vi "Apply.vi"(8 "error in":errorcluster, 11 "Camera Config Imaqdx in":refnum<class "Camera Imaqdx CFG.lvclass">) -> (0 "error out":errorcluster, 3 "Camera Config Imaqdx out":refnum<class "Camera Imaqdx CFG.lvclass">)   [LabVIEW 2023, in "Camera Imaqdx CFG.lvclass"]
uses:
  Camera Imaqdx CFG.lvclass
  Camera Imaqdx CFG.lvclass/Camera Imaqdx CFG.ctl
  <resource>/objmgr/imaqdx.rc
  <vilib>/vision/driver/IMAQdx.llb/IMAQdx Attribute Type.ctl
  c47df427-a957-40c2-9a9c-b1ab8804aafe.vi
  c5374de2-410c-459e-aecd-e99eee27f195.vi
  8bc8691d-3ecb-4910-bc1f-a4c379582725.vi
  7010e766-7afd-408f-98f0-f2143d80f09c.vi
  90c98f4d-8272-4d06-bdee-effaadf9e15a.vi
  4e38bbe0-b2bb-4691-89cd-49c1504e38ab.vi
  Configuration Base/Configuration Base.lvclass
  <vilib>/ErrorRing/Error Ring.xnode
  <vilib>/Utility/error.llb/Error Cluster From Error Code.vi
  E:/git/HAL/Configuration Base/Configuration Base.lvclass
  E:/git/HAL/Interfaces/IConfigure/IConfigure.lvclass
  E:/git/HAL/Camera Imaqdx/Configuration/Camera Imaqdx CFG.lvclass
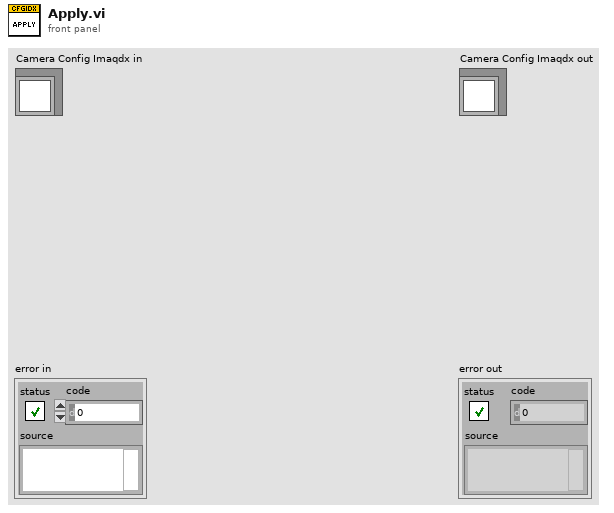
[diagram p1: front panel]
types:
  T1 = typedef "NI_Vision_Acquisition_Software.lvlib/IMAQdx Attribute Type.ctl" = enum32{"U32", "I64", "DBL", "String", "Enum", "Bool", "Command"}
  T2 = typedef "IMAQdx.ctl" = refnum<k21>
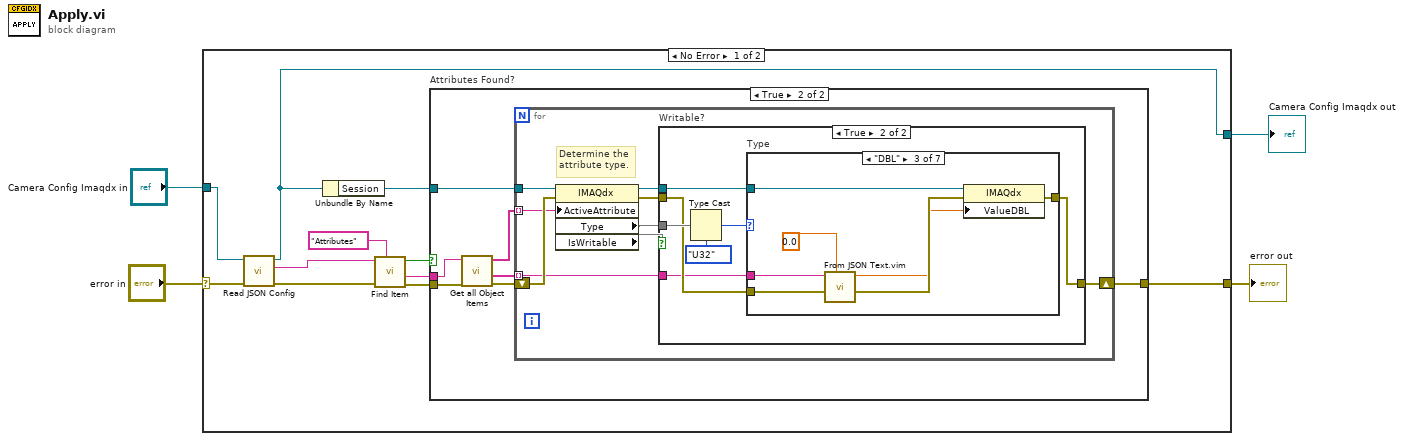
[diagram p0: block diagram]
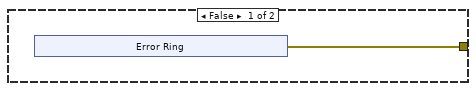
[diagram p2: hidden frame]
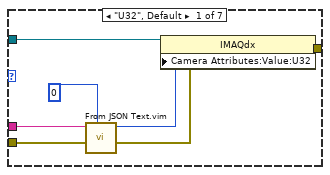
[diagram p4: hidden frame]
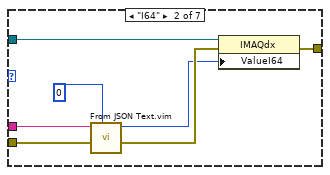
[diagram p5: hidden frame]
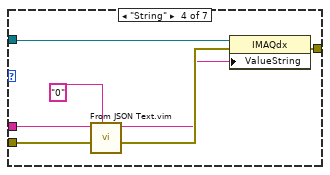
[diagram p6: hidden frame]
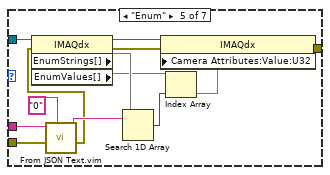
[diagram p7: hidden frame]
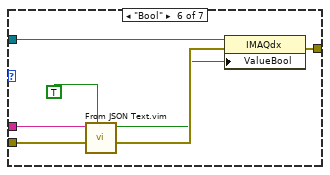
[diagram p8: hidden frame]
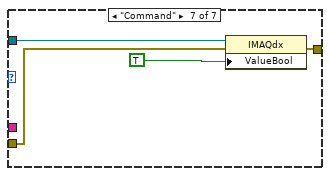
[diagram p9: hidden frame]
diagram:
  n1 = case shown="No Error" "error in" {
    selector: "error in" -> [w14 w98]
    tunnel: "Camera Config Imaqdx in" -> [w12 w99]
    tunnel: [w13 w98] -> w2
    tunnel: [w11 w99] -> w1
    frame No Error {
      n2 = call "Read JSON Config.vi"("error in (no error)"=w14, "Camera Config in"=w12) -> ("error out"=w10:errorcluster, "<JSON>Config"=w8:string, "Camera Config out"=w11:refnum<class "Camera Imaqdx CFG.lvclass">)  [unwired: 7 in]
      n3 = Unbundle By Name(w11) -> ("Session"=w15:T2)
      n4 = call <vilib>:"Find Item.vi"("$Path or Item Name"="Attributes", "error in (no error)"=w10, "JSON"=w8) -> ("error out"=w9:errorcluster, "<JSON>"=w6:string, "Found"=w5:bool)  [unwired: 5 in, 1 out]
      n5 = case "Attributes Found?" shown="True" w5 {
        tunnel: w15 -> [_ w28]
        tunnel: [w16 w24] -> w13
        tunnel: w9 -> [_ w23]
        tunnel: w6 -> [_ w22]
        frame False {
          n6 = xnode "Error Ring"() -> ("error out"=w16:errorcluster)
        }
        frame True {
          n7 = call <vilib>:"Get all Object Items.vi"("error in (no error)"=w23, "JSON"=w22) -> ("error out"=w27:errorcluster, "<JSON>"=w25:string[], "Item Names"=w26:string[])  [unwired: 6 in, 1 out]
          n8 = for {
            tunnel: w28 -> [w37]
            shift-right: [w30] -> w24
            shift-left: w27 -> [w36]
            tunnel: w26 -> [w35] mode=indexing
            tunnel: w25 -> [w31] mode=indexing
            # "Determine the\nattribute type."
            n9 = property class="IMAQdx"(reference=w37, error in=w36, "ActiveAttribute"=w35) -> (reference out=w32:T2, error out=w33:errorcluster, "Type"=w34, "IsWritable"=w29)
            n10 = case "Writable?" shown="True" w29 {
              tunnel: w34 -> [_ w44]
              tunnel: w33 -> [w38 w42]
              tunnel: w32 -> [_ w41]
              tunnel: w31 -> [_ w40]
              tunnel: [w38 w39] -> w30
              frame False {
              }
              frame True {
                n11 = Type Cast(type=IMAQdx_Attribute_Type."U32" ("Attribute Type"), x=w44) -> (*(type *) &x=w43:T1)
                n12 = case "Type" shown="\"DBL\"" w43 {
                  tunnel: w42 -> [w51 w54 w61 w67 w81 w87 w97]
                  tunnel: w41 -> [w52 w56 w63 w69 w83 w89 w95]
                  tunnel: w40 -> [w50 w55 w62 w68 w84 w88 _]
                  tunnel: [w46 w53 w60 w70 w85 w90 w94] -> w39
                  frame "U32", Default {
                    n13 = call "From JSON Text.vim"("Data Type and Default Value"=u32 0, "error in (no error)"=w51, "JSON"=w50) -> ("error out"=w49:errorcluster, "Data out"=w47:u32)  [unwired: 7 in]
                    n14 = property class="IMAQdx"(reference=w52, error in=w49, "Camera Attributes:Value:U32"=w47) -> (error out=w46:errorcluster)  [unwired: 1 out]
                  }
                  frame "I64" {
                    n15 = call "From JSON Text.vim"("Data Type and Default Value"=i64 0, "error in (no error)"=w54, "JSON"=w55) -> ("error out"=w59:errorcluster, "Data out"=w57:i64)  [unwired: 7 in]
                    n16 = property class="IMAQdx"(reference=w56, error in=w59, "ValueI64"=w57) -> (error out=w53:errorcluster)  [unwired: 1 out]
                  }
                  frame "DBL" {
                    n17 = call "From JSON Text.vim"("Data Type and Default Value"=0.0, "error in (no error)"=w61, "JSON"=w62) -> ("error out"=w66:errorcluster, "Data out"=w64:dbl)  [unwired: 7 in]
                    n18 = property class="IMAQdx"(reference=w63, error in=w66, "ValueDBL"=w64) -> (error out=w60:errorcluster)  [unwired: 1 out]
                  }
                  frame "String" {
                    n19 = call "From JSON Text.vim"("Data Type and Default Value"="0", "error in (no error)"=w67, "JSON"=w68) -> ("error out"=w73:errorcluster, "Data out"=w71:string)  [unwired: 7 in]
                    n20 = property class="IMAQdx"(reference=w69, error in=w73, "ValueString"=w71) -> (error out=w70:errorcluster)  [unwired: 1 out]
                  }
                  frame "Enum" {
                    n21 = call "From JSON Text.vim"("Data Type and Default Value"="0", "error in (no error)"=w81, "JSON"=w84) -> ("error out"=w75:errorcluster, "Data out"=w79:string)  [unwired: 7 in]
                    n22 = property class="IMAQdx"(reference=w83, error in=w75) -> (reference out=w82:T2, error out=w74:errorcluster, "EnumStrings[]"=w80, "EnumValues[]"=w77)
                    n23 = Search 1D Array(1D array=w80, element=w79) -> (index of element=w78:i32)  [unwired: 1 in]
                    n24 = Index Array(array=w77, index=w78) -> (element=w76)
                    n25 = property class="IMAQdx"(reference=w82, error in=w74, "Camera Attributes:Value:U32"=w76) -> (error out=w85:errorcluster)  [unwired: 1 out]
                  }
                  frame "Bool" {
                    n26 = call "From JSON Text.vim"("Data Type and Default Value"=TRUE, "error in (no error)"=w87, "JSON"=w88) -> ("error out"=w93:errorcluster, "Data out"=w91:bool)  [unwired: 7 in]
                    n27 = property class="IMAQdx"(reference=w89, error in=w93, "ValueBool"=w91) -> (error out=w90:errorcluster)  [unwired: 1 out]
                  }
                  frame "Command" {
                    n28 = property class="IMAQdx"(reference=w95, error in=w97, "ValueBool"=TRUE) -> (error out=w94:errorcluster)  [unwired: 1 out]
                  }
                }
              }
            }
          }
        }
      }
    }
    frame Error {
    }
  }
  "error out" <- w2
  "Camera Config Imaqdx out" <- w1
